vi "Configure Sequencer List All Dwell Times.vi"(7 "Dwell Times":dbl[](array[numeric]) format="%^.3e", 8 "error in (no error)":errorcluster, 10 "Instance (1)":i32=1, 11 "VISA resource name":refnum<visa-resource-name>) -> (0 "error out":errorcluster, 3 "VISA resource name out":refnum<visa-resource-name>)   [LabVIEW 2015, in "Rohde&Schwarz CMXP GPRF.lvlib"]
doc: "Defines the dwell times for all sequencer list entries.\n\nAttribute:\nRSCMXPGPRF_ATTR_SEQUENCER_LIST_ALL_DWELL_TIMES\n\nRemote-control command:\nSOURce:GPRF:GEN<i>:SEQuencer:LIST:DTIMe:ALL"
uses:
  <instrlib>/Rohde&Schwarz CMXP GPRF/Rohde&Schwarz CMXP GPRF.lvlib
  <instrlib>/Rohde&Schwarz CMXP GPRF/Private/rsidr_core.llb/rsidr_core.lvlib
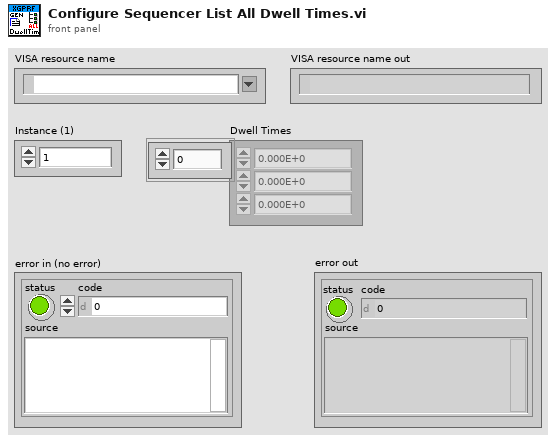
[diagram p1: front panel]
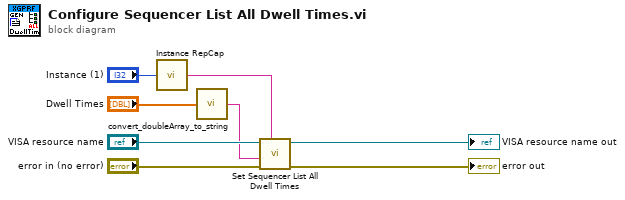
[diagram p0: block diagram]
diagram:
  n1 = call <instrlib>:"Instance RepCap.vi"("instance  in"="Instance (1)") -> ("instance out"=w5:string)
  n2 = call <instrlib>:"convert_doubleArray_to_string.vi"("double array in"="Dwell Times") -> ("string out"=w1:string)  [unwired: 4 in]
  n3 = call "Set Sequencer List All Dwell Times"("Repeated Capabilities"=w5, "error in (no error)"="error in (no error)", "Sequencer List All Dwell Times ()"=w1, "instrument handle"="VISA resource name") -> ("error out"=→"error out":errorcluster, "instrument handle out"=→"VISA resource name out":refnum<visa-resource-name>)  [unwired: 6 in]
